vi "Convert Unicode to Big5.vi"(10 "UNICODEString":string) -> (2 "Big5String":string)   [LabVIEW 2013]
uses:
  <vilib>/Utility/file.llb/Read From Spreadsheet File (string).vi
  <vilib>/regexp/Match Regular Expression.xnode
panel:
  in  "file path (dialog if empty)":path=path "C:/Users/cleo/Desktop/unicode/cp950-u2b.txt"
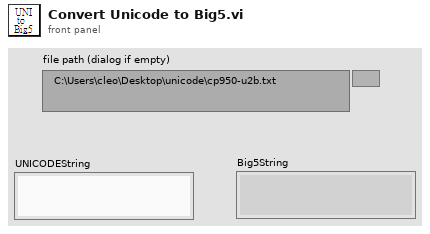
[diagram p1: front panel]
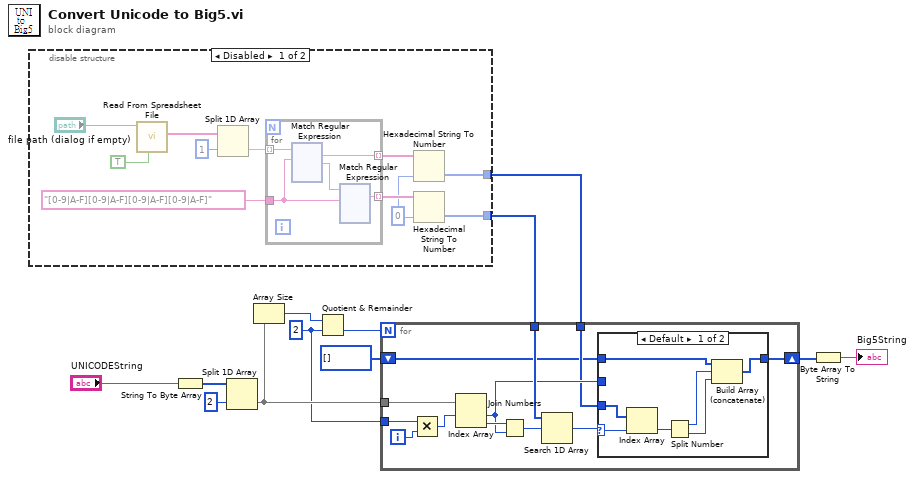
[diagram p0: block diagram]
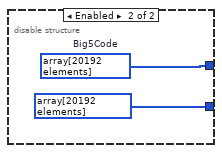
[diagram p2: hidden frame]
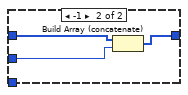
[diagram p3: hidden frame]
diagram:
  w6 = 2 ("y")
  n1 = disable-structure shown="Disabled" {
    disable-tunnel: [w14 u16[] array[20192 elements] ("UniCODE")] -> w5
    disable-tunnel: [w13 w258] -> w4
    frame Disabled {
      w15 = u16 0 ("default (0 U32)")
      n2 = call-poly <vilib>:"Read From Spreadsheet File.vi"("transpose (no:F)"=TRUE, "file path (dialog if empty)"="file path (dialog if empty)") -> ("first row"=w21:string[])  [unwired: 5 in, 4 out]
      n3 = Split 1D Array(array=w21, index=1) -> (second subarray=w18:string[])  [unwired: 1 out]
      n4 = for {
        tunnel: "[0-9|A-F][0-9|A-F][0-9|A-F][0-9|A-F]" ("regular expression") -> [w27]
        tunnel: w18 -> [w26] mode=indexing
        tunnel: [w25] -> w17 mode=indexing
        tunnel: [w24] -> w16 mode=indexing
        n5 = xnode "Match Regular Expression"("input string"=w26, "regular expression"=w27) -> ("whole match"=w25:string, "after match"=w28:string)  [unwired: 4 in, 3 out]
        n6 = xnode "Match Regular Expression"("input string"=w28, "regular expression"=w27) -> ("whole match"=w24:string)  [unwired: 4 in, 4 out]
      }
      n7 = Hexadecimal String To Number(string=w17, default (0uL)=w15) -> (number=w13:u16[])  [unwired: 1 in, 1 out]
      n8 = Hexadecimal String To Number(string=w16, default (0uL)=w15) -> (number=w14:u16[])  [unwired: 1 in, 1 out]
    }
    frame Enabled {
      w258 = u16[] array[20192 elements]  # Big5Code
    }
  }
  n9 = String To Byte Array(string="UNICODEString") -> (unsigned byte array=w11:u8[])
  n10 = Split 1D Array(array=w11, index=2) -> (second subarray=w7:u8[])  [unwired: 1 out]
  n11 = Array Size(array=w7) -> (size(s)=w9:i32)
  n12 = Quotient & Remainder(x=w9, y=w6) -> (floor(x/y)=w8:i32)  [unwired: 1 out]
  n13 = for {
    N: w8 -> [_]
    tunnel: w7 -> [w270]
    tunnel: w6 -> [w269]
    tunnel: w5 -> [w265]
    tunnel: w4 -> [w261]
    shift-right: [w260] -> w2
    shift-left: u8[] [] -> [w259]
    i -> [w268]
    n14 = Multiply(x=w269, y=w268) -> (x*y=w267:i32)
    n15 = Index Array(array=w270, index #1=w267) -> (element #1=w262:u8, element #2=w266:u8)  [unwired: 1 in]
    n16 = Join Numbers(hi=w266, lo=w262) -> ((hi.lo)=w264:u16)
    n17 = Search 1D Array(1D array=w265, element=w264) -> (index of element=w263:i32)  [unwired: 1 in]
    n18 = case shown="Default" w263 {
      selector: w263 -> [w277 _]
      tunnel: w262 -> [_ w279]
      tunnel: w261 -> [w276 _]
      tunnel: [w272 w278] -> w260
      tunnel: w259 -> [w271 w280]
      frame Default {
        n19 = Index Array(array=w276, index=w277) -> (element=w275:u16)
        n20 = Split Number(x=w275) -> (hi(x)=w274:u8, lo(x)=w273:u8)
        n21 = Build Array (concatenate)(w271, w274, w273) -> (w272:u8[])
      }
      frame -1 {
        n22 = Build Array (concatenate)(w280, w279) -> (w278:u8[])
      }
    }
  }
  n23 = Byte Array To String(unsigned byte array=w2) -> (string=→"Big5String":string)
